vi "Write Roles.vi"(8 "error in (no error)":errorcluster, 10 "Role":T1, 11 "PassTo2ndStriker in":refnum<class "PassTo2ndStriker.lvclass">) -> (0 "error out":errorcluster, 3 "PassTo2ndStriker out":refnum<class "PassTo2ndStriker.lvclass">)   [LabVIEW 2023, in "PassTo2ndStriker.lvclass"]
uses:
  PassTo2ndStriker.lvclass
  PassKickerRole_class/PassKickerRole.lvclass
  PassReceiverRole_class/PassReceiverRole.lvclass
  PassObserverRole_class/PassObserverRole.lvclass
  PassTo2ndStriker.lvclass/PassTo2ndStriker.ctl
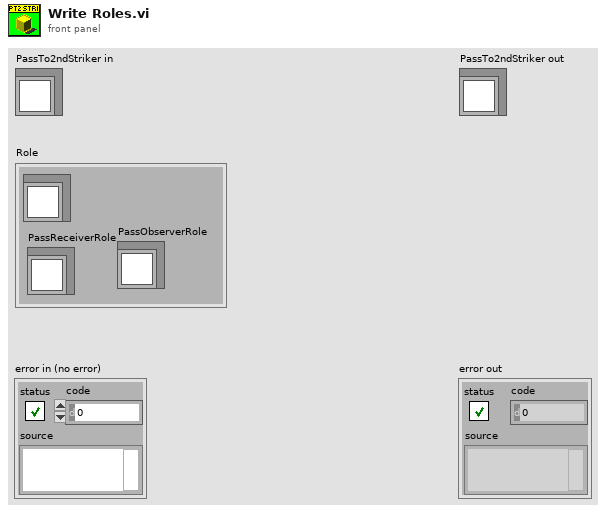
[diagram p1: front panel]
types:
  T1 = cluster{"PassKickerRole":refnum<class "PassKickerRole.lvclass">, "PassReceiverRole":refnum<class "PassReceiverRole.lvclass">, "PassObserverRole":refnum<class "PassObserverRole.lvclass">}
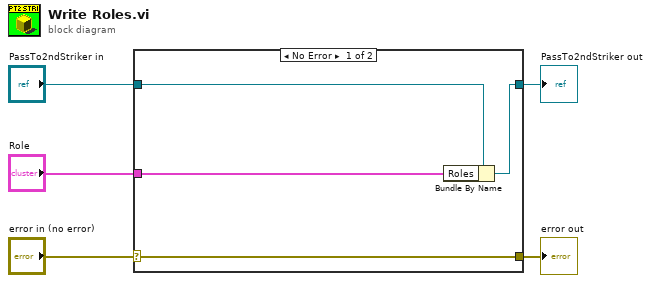
[diagram p0: block diagram]
diagram:
  n1 = case shown="No Error" "error in (no error)" {
    selector: "error in (no error)" -> [w9 w10]
    tunnel: [w9 w10] -> w4
    tunnel: [w7 w11] -> w2
    tunnel: "PassTo2ndStriker in" -> [w8 w11]
    tunnel: "Role" -> [w6 _]
    frame No Error {
      n2 = Bundle By Name(cluster=w8, "Roles"=w6) -> (w7:refnum<class "PassTo2ndStriker.lvclass">)
    }
    frame Error {
    }
  }
  "error out" <- w4
  "PassTo2ndStriker out" <- w2
